vi "Actor Core.vi"(8 "error in":errorcluster, 11 "Target in":refnum<class "Target.lvclass">) -> (0 "error out":errorcluster, 3 "Actor out":refnum<class "Actor.lvclass">)   [LabVIEW 2014, in "Target.lvlib" / "Target.lvclass"]
doc: "(<B>Filename</B>: Actor Framework.lvlib:Actor.lvclass:Actor Core.vi)\n\nReceives messages to the actor, reacts to them, and initiates any error handling that may shut the actor down.\n\nDescendant classes may override this VI to append parallel tasks for the actor to complete while it handles messages. Overrides use the Call Parent Method node."
uses:
  Target.lvclass
  <vilib>/ActorFramework/Actor/Actor.lvclass
  Proxy/Proxy/Proxy.lvclass
  Target.lvclass/Target.ctl
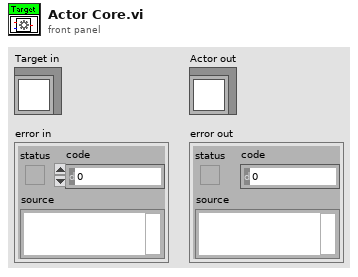
[diagram p1: front panel]
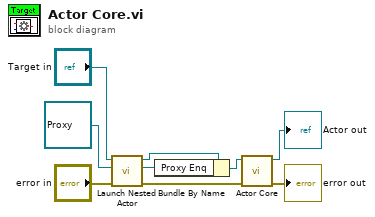
[diagram p0: block diagram]
diagram:
  n1 = call <vilib>:"Launch Nested Actor.vi"("error in (no error)"="error in", "Nested Actor"=refnum<class "Proxy.lvclass"> refnum ("Proxy.lvlib:Proxy.lvclass"), "Caller Actor in"="Target in") -> ("error out"=w3:errorcluster, "Nested Actor's Enqueuer"=w1:refnum<class "Message Enqueuer.lvclass">, "Caller Actor out"=w5:refnum<class "Target.lvclass">)  [unwired: 6 in]
  n2 = Bundle By Name(cluster=w5, "Proxy Enq"=w1) -> (w2:refnum<class "Target.lvclass">)
  n3 = call-parent "Actor Core.vi"("error in"=w3, "Actor in"=w2) -> ("error out"=→"error out":errorcluster, "Actor out"=→"Actor out":refnum<class "Actor.lvclass">)  [unwired: 8 in]
